vi "현재시간(SubVI).vi"() -> (0 "시간 숫자":i32, 1 "시간 문자열":string, 2 "분":i32, 3 "시":i32, 4 "분 문자열":string, 5 "날짜/시간 문자열":string, 6 "시 문자열":string, 8 "초":i32, 9 "초 문자열":string)   [LabVIEW 2014]
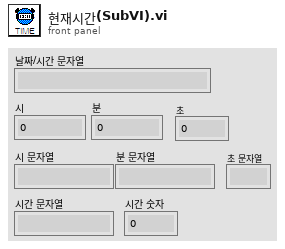
[diagram p1: front panel]
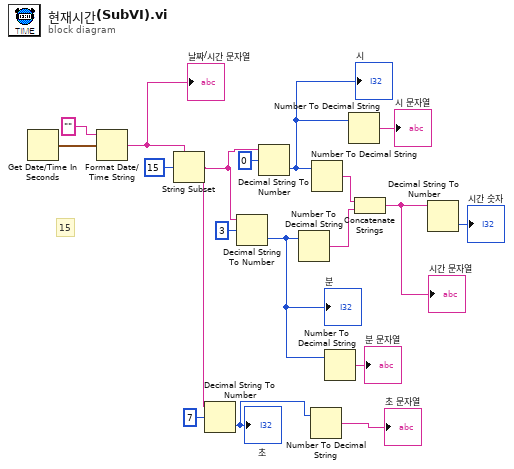
[diagram p0: block diagram]
diagram:
  # "15"
  n1 = Get Date/Time In Seconds() -> (seconds since 1Jan1904=w13:timestamp)
  n2 = Format Date/Time String(time format string (%c)="" ("시간 포맷 문자열 (%c)"), seconds (now)=w13) -> (date/time string=w1:string)  [unwired: 1 in]
  "날짜/시간 문자열" <- w1
  n3 = String Subset(string=w1, offset (0)=15 ("오프셋(0)")) -> (substring=w2:string)  [unwired: 1 in]
  n4 = Decimal String To Number(string=w2, offset=7 ("오프셋")) -> (number=w4:i32)  [unwired: 1 in, 1 out]
  "초" <- w4
  n5 = Decimal String To Number(string=w2, offset=3 ("오프셋")) -> (number=w7:i32)  [unwired: 1 in, 1 out]
  "분" <- w7
  n6 = Decimal String To Number(string=w2, offset=0 ("오프셋")) -> (number=w9:i32)  [unwired: 1 in, 1 out]
  "시" <- w9
  n7 = Number To Decimal String(number=w7) -> (decimal integer string=w18:string)  [unwired: 1 in]
  n8 = Number To Decimal String(number=w4) -> (decimal integer string=→"초 문자열":string)  [unwired: 1 in]
  n9 = Number To Decimal String(number=w9) -> (decimal integer string=w17:string)  [unwired: 1 in]
  n10 = Number To Decimal String(number=w7) -> (decimal integer string=→"분 문자열":string)  [unwired: 1 in]
  n11 = Number To Decimal String(number=w9) -> (decimal integer string=→"시 문자열":string)  [unwired: 1 in]
  n12 = Concatenate Strings(w17, w18) -> (w11:string)
  "시간 문자열" <- w11
  n13 = Decimal String To Number(string=w11) -> (number=→"시간 숫자":i32)  [unwired: 2 in, 1 out]
